vi "Display Float Values As Graph.vi"() -> ()   [LabVIEW 2014]
panel:
  out "Waveform Graph 2":dbl[](graph)
  out "Waveform Graph":dbl[](graph)
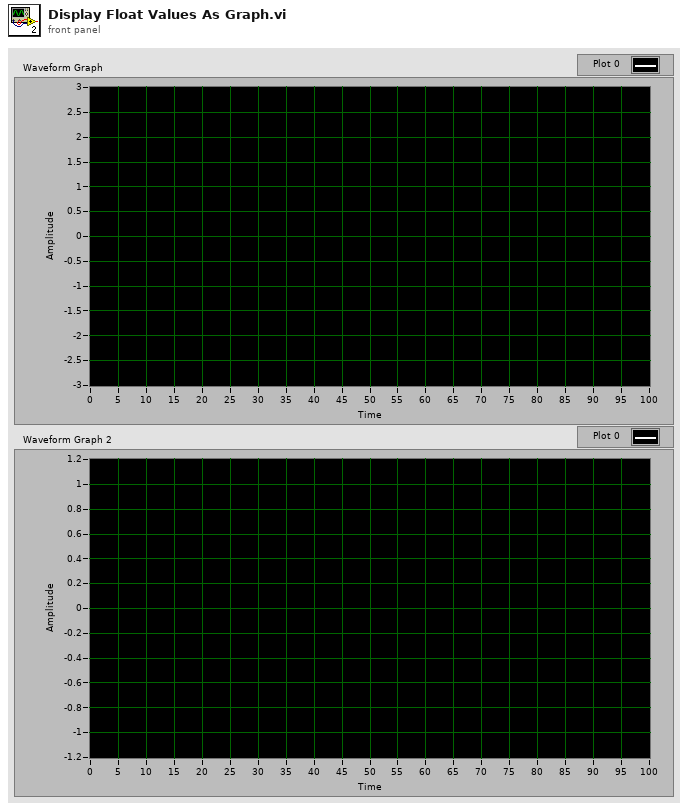
[diagram p1: front panel]
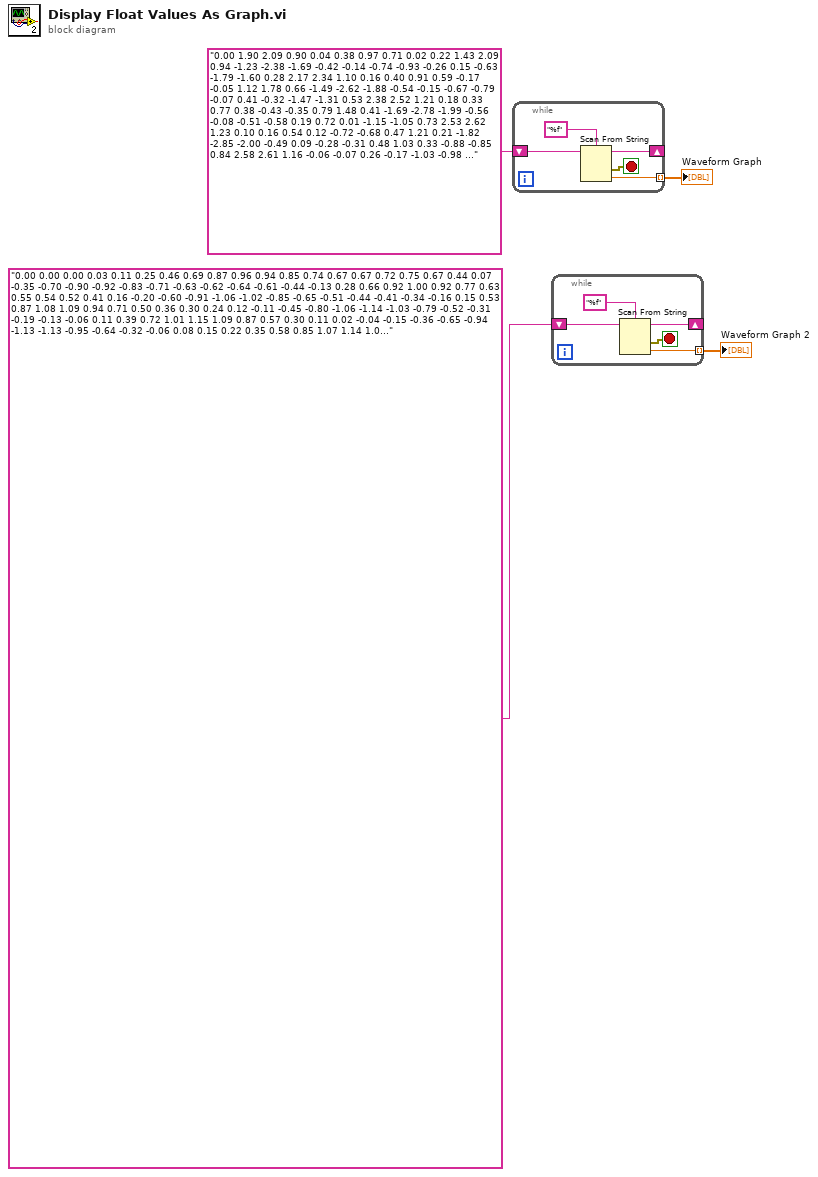
[diagram p0: block diagram]
diagram:
  n1 = while {
    shift-right: [w7] -> _
    shift-left: "0.00 1.90 2.09 0.90 0.04 0.38 0.97 0.71 0.02 0.22 1.43 2.09 0.94 -1.23 -2.38 -1.69 -0.42 -0.14 -0.74 -0.93 -0.26 0.15 -0.63 -1.79 -1.60 0.28 2.17 2.34 1.10 0.16 0.40 0.91 0.59 -0.17 -0.05 1.12 1.78 0.66 -1.49 -2.62 -1.88 -0.54 -0.15 -0.67 -0.79 -0.07 0.41 -0.32 -1.47 -1.31 0.53 2.38 2.52 1.21 0.18 0.33 0.77 0.38 -0.43 -0.35 0.79 1.48 0.41 -1.69 -2.78 -1.99 -0.56 -0.08 -0.51 -0.58 0.19 0.72 0.01 -1.15 -1.05 0.73 2.53 2.62 1.23 0.10 0.16 0.54 0.12 -0.72 -0.68 0.47 1.21 0.21 -1.82 -2.85 -2.00 -0.49 0.09 -0.28 -0.31 0.48 1.03 0.33 -0.88 -0.85 0.84 2.58 2.61 1.16 -0.06 -0.07 0.26 -0.17 -1.03 -0.98 0.19 1.01 0.10 -1.85 -2.83 -1.92 -0.33 0.32 0.01 -0.01 0.78 1.32 0.60 -0.67 -0.73 0.87 2.54 2.52 1.00 -0.29 -0.36 -0.04 -0.47 -1.31 -1.25 -0.02 0.88 0.07 -1.80 -2.72 -1.75 -0.10 0.61 0.32 0.29 1.06 1.57 0.81 -0.54 -0.70 0.80 2.41 2.34 0.77 -0.57 -0.68 -0.35 -0.75 -1.55 -1.44 -0.15 0.85 0.14 -1.65 -2.52 -1.52 0.18 0.92 0.63 0.57 1.29 1.75 0.93 -0.50 -0.77 0.64 2.19 2.09 0.49 -0.88 -0.99 -0.64 -0.97 -1.72 -1.55 -0.19 0.91 0.30 -1.42 -2.26 -1.24 0.47 1.23 0.92 0.80 1.44 1.84 0.96 -0.56 -0.93 0.41 1.91 1.80 0.20 -1.17 -1.27 -0.86 -1.12 -1.79 -1.56 -0.13 1.06 0.54 -1.12 -1.96 -0.95 0.76 1.50 1.14 0.95 1.51 1.84 0.89 -0.70 -1.16 0.11 1.60 1.50 -0.07 -1.43 -1.49 -1.01 -1.19 -1.78 -1.48 0.02 1.28 0.84 -0.80 -1.64 -0.67 1.00 1.70 1.29 1.01 1.48 1.75 0.73 -0.92 -1.45 -0.22 1.27 1.22 -0.31 -1.62 -1.63 -1.07 -1.15 -1.67 -1.31 0.24 1.56 1.16 -0.47 -1.35 -0.44 1.18 1.83 1.34 0.97 1.36 1.56 0.51 -1.19 -1.76 -0.55 0.97 0.99 -0.48 -1.73 -1.68 -1.03 -1.03 -1.47 -1.08 0.51 1.86 1.49 -0.16 -1.11 -0.28 1.28 1.87 1.30 0.84 1.16 1.31 0.24 -1.48 -2.07 -0.86 0.72 0.82 -0.56 -1.75 -1.63 -0.91 -0.82 -1.21 -0.80 0.80 2.16 1.79 0.10 -0.93 -0.19 1.28 1.80 1.17 0.64 0.89 1.02 -0.05 -1.77 -2.36 -1.11 0.54 0.74 -0.56 -1.67 -1.49 -0.70 -0.55 -0.91 -0.50 1.08 2.43 2.03 0.28 -0.84 -0.21 1.19 1.65 0.96 0.37 0.58 0.71 -0.34 -2.02 -2.58 -1.29 0.44 0.75 -0.45 -1.51 -1.27 -0.43 -0.24 -0.59 -0.21 1.32 2.64 2.19 0.37 -0.85 -0.32 1.01 1.43 0.70 0.06 0.26 0.42 -0.58 -2.22 -2.73 -1.38 0.45 0.85 -0.26 -1.27 -1.00 -0.13 0.08 -0.29 0.03 1.50 2.76 2.27 0.37 -0.95 -0.51 0.75 1.15 0.40 -0.25 -0.04 0.17 -0.76 -2.33 -2.79 -1.37 0.54 1.05 0.00 -0.97 -0.70 0.17 0.37 -0.04 0.22 1.60 2.80 2.25 0.28 -1.14 -0.77 0.45 0.84 0.10 -0.53 -0.29 -0.01 -0.85 -2.35 -2.75 -1.27 0.72 1.30 0.31 -0.66 -0.40 0.44 0.61 0.15 0.31 1.61 2.74 2.13 0.10 -1.39 -1.08 0.13 0.54 -0.17 -0.76 -0.47 -0.11 -0.86 -2.27 -2.61 -1.09 0.96 1.61 0.64 -0.35 -0.14 0.67 0.79 0.25 0.32 1.52 2.59 1.94 -0.14 -1.68 -1.41 -0.19 0.26 -0.38 -0.93 -0.56 -0.12 -0.76 -2.10 -2.40 -0.85 1.24 1.92 0.96 -0.07 0.08 0.82 0.87 0.25 0.22 1.35 2.36 1.69 -0.41 -1.98 -1.72 -0.47 0.05 -0.52 -1.00 -0.56 -0.03 -0.58 -1.86 -2.13 -0.57 1.53 2.22 1.24 0.15 0.21 0.87 0.86 0.16 0.04 1.09 2.07 1.40 -0.70 -2.27 -2.00 -0.69 -0.09 -0.57 -0.97 -0.47 0.15 -0.33 -1.56 -1.84 -0.29 1.81 2.48 1.45 0.29 0.26 0.84 0.76 -0.02 -0.21 0.79 1.76 1.11 -0.96 -2.51 -2.20 -0.83 -0.13 -0.52 -0.86 -0.29 0.39 -0.03 -1.24 -1.53 -0.03 2.03 2.68 1.59 0.33 0.20 0.71 0.57 -0.26 -0.50 0.46 1.45 0.85 -1.17 -2.69 -2.33 -0.88 -0.08 -0.39 -0.66 -0.04 0.68 0.30 -0.92 -1.26 0.19 2.19 2.78 1.63 0.28 0.06 0.50 0.32 -0.55 -0.82 0.14 1.16 0.63 -1.32 -2.77 -2.36 -0.83 0.07 -0.17 -0.39 0.24 0.99 0.62 -0.63 -1.04 0.32 2.26 2.80 1.58 0.14 -0.16 0.23 0.02 -0.85 -1.13 -0.15 0.94 0.49 -1.37 -2.77 -2.29 -0.69 0.28 0.11 -0.09 0.54 1.29 0.90 -0.40 -0.89 0.37 2.23 2.71 1.43 -0.07 -0.44 -0.08 -0.28 -1.14 -1.40 -0.38 0.78 0.44 -1.33 -2.66 -2.14 -0.47 0.56 0.42 0.22 0.83 1.55 1.12 -0.24 -0.84 0.33 2.11 2.54 1.22 -0.34 -0.75 -0.40 -0.57 -1.38 -1.60 -0.53 0.72 0.49 -1.20 -2.48 -1.91 -0.21 0.86 0.74 0.51 1.07 1.74 1.26 -0.18 -0.88 0.19 1.91 2.30 0.95 -0.64 -1.06 -0.69 -0.81 -1.56 -1.73 -0.58 0.76 0.63 -0.98 -2.22 -1.64 0.08 1.17 1.03 0.75 1.24 1.85 1.30 -0.21 -1.01 -0.03 1.63 2.02 0.66 -0.93 -1.35 -0.93 -0.98 -1.66 -1.76 -0.54 0.89 0.84 -0.70 -1.92 -1.35 0.37 1.44 1.27 0.92 1.33 1.86 1.25 -0.34 -1.22 -0.32 1.32 1.71 0.38 -1.20 -1.58 -1.10 -1.06 -1.66 -1.69 -0.42 1.09 1.12 -0.38 -1.60 -1.06 0.62 1.66 1.44 1.00 1.32 1.78 1.11 -0.54 -1.49 -0.64 0.99 1.42 0.13 -1.40 -1.73 -1.18 -1.05 -1.57 -1.54 -0.21 1.35 1.44 -0.04 -1.29 -0.81 0.81 1.80 1.51 0.99 1.22 1.61 0.90 -0.80 -1.80 -0.97 0.68 1.16 -0.05 -1.53 -1.80 -1.17 -0.95 -1.38 -1.31 0.05 1.65 1.76 0.28 -1.03 -0.63 0.92 1.85 1.49 0.88 1.03 1.37 0.63 -1.08 -2.11 -1.29 0.41 0.97 -0.16 -1.56 -1.77 -1.06 -0.76 -1.13 -1.03 0.34 1.94 2.06 0.55 -0.83 -0.52 0.94 1.81 1.38 0.70 0.78 1.08 0.34 -1.37 -2.39 -1.55 0.20 0.87 -0.17 -1.50 -1.65 -0.87 -0.50 -0.83 -0.73 0.62 2.21 2.31 0.75 -0.72 -0.51 0.87 1.67 1.19 0.44 0.48 0.77 0.05 -1.63 -2.63 -1.74 0.08 0.85 -0.09 -1.35 -1.44 -0.62 -0.20 -0.52 -0.43 0.88 2.43 2.49 0.86 -0.70 -0.60 0.70 1.46 0.93 0.15 0.16 0.46 -0.21 -1.84 -2.78 -1.85 0.06 0.93 0.09 -1.12 -1.18 -0.33 0.11 -0.21 -0.17 1.07 2.57 2.58 0.89 -0.77 -0.77 0.46 1.18 0.64 -0.16 -0.15 0.20 -0.41 -1.96 -2.85 -1.86 0.13 1.10 0.33 -0.83 -0.88 -0.03 0.41 0.06 0.03 1.19 2.62 2.58 0.81 -0.93 -1.02 0.16 0.87 0.34 -0.45 -0.41 -0.01 -0.52 -2.00 -2.83 -1.78 0.29 1.34 0.64 -0.51 -0.58 0.25 0.66 0.26 0.15 1.22 2.58 2.48 0.65 -1.16 -1.31 -0.16 0.56 0.06 -0.69 -0.61 -0.13 -0.55 -1.94 -2.71 -1.61 0.51 1.63 0.96 -0.19 -0.30 0.49 0.85 0.38 0.18 1.15 2.44 2.29 0.43 -1.44 -1.63 -0.48 0.28 -0.17 -0.87 -0.72 -0.16 -0.48 -1.79 -2.51 -1.38 0.79 1.94 1.28 0.10 -0.07 0.65 0.95 0.41 0.11 1.00 2.22 2.04 0.16 -1.74 -1.95 -0.78 0.04 -0.33 -0.96 -0.74 -0.09 -0.32 -1.56 -2.24 -1.10 1.07 2.24 1.57 0.34 0.09 0.73 0.96 0.34 -0.05 0.76 1.94 1.76 -0.13 -2.03 -2.23 -1.02 -0.12 -0.40 -0.95 -0.66 0.06 -0.09 -1.27 -1.94 -0.81 1.35 2.50 1.81 0.50 0.15 0.71 0.87 0.18 -0.28 0.47 1.62 1.46 -0.40 -2.28 -2.45 -1.18 -0.18 -0.37 -0.85 -0.50 0.29 0.20 -0.94 -1.63 -0.54 1.58 2.71 1.96 0.57 0.13 0.60 0.70 -0.05 -0.56 0.14 1.30 1.18 -0.62 -2.46 -2.59 -1.24 -0.16 -0.25 -0.66 -0.27 0.57 0.52 -0.62 -1.34 -0.32 1.75 2.83 2.02 0.54 0.01 0.40 0.46 -0.32 -0.87 -0.18 1.01 0.95 -0.78 -2.56 -2.63 -1.22 -0.04 -0.05 -0.41 0.02 0.87 0.84 -0.32 -1.10 -0.16 1.83 2.85 1.98 0.42 -0.20 0.14 0.17 -0.63 -1.18 -0.48 0.76 0.79 -0.86 -2.57 -2.58 -1.10 0.16 0.22 -0.11 0.32 1.17 1.13 -0.07 -0.93 -0.09 1.83 2.79 1.86 0.23 -0.46 -0.16 -0.14 -0.92 -1.46 -0.72 0.58 0.71 -0.84 -2.48 -2.44 -0.90 0.42 0.52 0.20 0.61 1.44 1.36 0.11 -0.85 -0.11 1.72 2.63 1.66 -0.03 -0.77 -0.48 -0.44 -1.17 -1.67 -0.89 0.50 0.73 -0.72 -2.30 -2.23 -0.65 0.72 0.84 0.50 0.86 1.64 1.51 0.19 -0.86 -0.22 1.53 2.39 1.40 -0.32 -1.08 -0.78 -0.69 -1.37 -1.81 -0.96 0.51 0.84 -0.52 -2.05 -1.96 -0.36 1.02 1.14 0.76 1.05 1.76 1.57 0.18 -0.97" -> [w9]
    tunnel: [w5] -> w3 mode=indexing
    stop <- w6 stop-if-true
    n2 = Scan From String(format string="%f", input string=w9) -> (remaining string=w7:string, error out=w6:errorcluster, output 1=w5:dbl)  [unwired: 3 in, 1 out]
  }
  "Waveform Graph" <- w3
  n3 = while {
    shift-right: [w12] -> _
    shift-left: "0.00 0.00 0.00 0.03 0.11 0.25 0.46 0.69 0.87 0.96 0.94 0.85 0.74 0.67 0.67 0.72 0.75 0.67 0.44 0.07 -0.35 -0.70 -0.90 -0.92 -0.83 -0.71 -0.63 -0.62 -0.64 -0.61 -0.44 -0.13 0.28 0.66 0.92 1.00 0.92 0.77 0.63 0.55 0.54 0.52 0.41 0.16 -0.20 -0.60 -0.91 -1.06 -1.02 -0.85 -0.65 -0.51 -0.44 -0.41 -0.34 -0.16 0.15 0.53 0.87 1.08 1.09 0.94 0.71 0.50 0.36 0.30 0.24 0.12 -0.11 -0.45 -0.80 -1.06 -1.14 -1.03 -0.79 -0.52 -0.31 -0.19 -0.13 -0.06 0.11 0.39 0.72 1.01 1.15 1.09 0.87 0.57 0.30 0.11 0.02 -0.04 -0.15 -0.36 -0.65 -0.94 -1.13 -1.13 -0.95 -0.64 -0.32 -0.06 0.08 0.15 0.22 0.35 0.58 0.85 1.07 1.14 1.01 0.72 0.36 0.05 -0.16 -0.26 -0.31 -0.38 -0.54 -0.77 -0.99 -1.11 -1.04 -0.79 -0.43 -0.06 0.22 0.37 0.42 0.45 0.53 0.70 0.90 1.04 1.04 0.85 0.50 0.11 -0.23 -0.45 -0.53 -0.54 -0.56 -0.65 -0.81 -0.96 -1.00 -0.87 -0.57 -0.17 0.22 0.50 0.63 0.64 0.62 0.64 0.73 0.86 0.93 0.86 0.62 0.24 -0.17 -0.51 -0.70 -0.75 -0.71 -0.66 -0.68 -0.76 -0.84 -0.82 -0.64 -0.31 0.11 0.49 0.75 0.85 0.81 0.72 0.66 0.68 0.73 0.75 0.63 0.36 -0.04 -0.45 -0.76 -0.92 -0.91 -0.80 -0.68 -0.62 -0.63 -0.65 -0.58 -0.38 -0.03 0.38 0.74 0.96 1.00 0.89 0.73 0.60 0.54 0.54 0.50 0.36 0.08 -0.31 -0.69 -0.96 -1.06 -0.99 -0.80 -0.61 -0.48 -0.43 -0.40 -0.31 -0.09 0.24 0.62 0.94 1.10 1.07 0.89 0.65 0.45 0.34 0.29 0.23 0.08 -0.19 -0.54 -0.88 -1.10 -1.13 -0.98 -0.72 -0.46 -0.27 -0.18 -0.12 -0.03 0.17 0.47 0.81 1.06 1.15 1.05 0.80 0.50 0.24 0.08 0.01 -0.06 -0.19 -0.42 -0.72 -1.00 -1.14 -1.10 -0.88 -0.56 -0.24 -0.01 0.10 0.16 0.24 0.40 0.65 0.92 1.10 1.12 0.95 0.64 0.28 -0.02 -0.20 -0.28 -0.32 -0.41 -0.59 -0.83 -1.03 -1.11 -0.99 -0.71 -0.34 0.02 0.27 0.39 0.42 0.46 0.57 0.75 0.95 1.06 1.01 0.77 0.41 0.01 -0.30 -0.48 -0.53 -0.54 -0.58 -0.69 -0.85 -0.98 -0.98 -0.81 -0.48 -0.07 0.30 0.54 0.64 0.64 0.62 0.66 0.77 0.89 0.93 0.82 0.54 0.14 -0.27 -0.58 -0.73 -0.74 -0.69 -0.66 -0.70 -0.79 -0.85 -0.79 -0.57 -0.21 0.21 0.57 0.79 0.85 0.78 0.70 0.66 0.69 0.74 0.73 0.58 0.27 -0.14 -0.54 -0.82 -0.93 -0.89 -0.76 -0.66 -0.62 -0.64 -0.64 -0.54 -0.30 0.07 0.48 0.81 0.99 0.98 0.85 0.69 0.58 0.54 0.53 0.48 0.30 -0.01 -0.40 -0.77 -1.01 -1.06 -0.95 -0.75 -0.57 -0.46 -0.42 -0.39 -0.27 -0.02 0.33 0.71 0.99 1.11 1.03 0.83 0.59 0.42 0.32 0.28 0.20 0.02 -0.27 -0.63 -0.95 -1.12 -1.11 -0.92 -0.65 -0.40 -0.24 -0.16 -0.10 0.02 0.24 0.56 0.88 1.10 1.15 1.00 0.72 0.42 0.19 0.06 -0.01 -0.08 -0.24 -0.49 -0.80 -1.05 -1.15 -1.06 -0.81 -0.47 -0.17 0.02 0.12 0.18 0.27 0.46 0.72 0.97 1.13 1.10 0.88 0.54 0.19 -0.08 -0.22 -0.29 -0.34 -0.45 -0.65 -0.89 -1.07 -1.10 -0.94 -0.62 -0.24 0.09 0.31 0.40 0.43 0.48 0.61 0.80 0.98 1.06 0.97 0.69 0.31 -0.08 -0.36 -0.50 -0.54 -0.54 -0.60 -0.73 -0.89 -1.00 -0.96 -0.74 -0.38 0.03 0.37 0.58 0.64 0.63 0.62 0.68 0.80 0.90 0.92 0.77 0.45 0.04 -0.36 -0.63 -0.74 -0.73 -0.68 -0.66 -0.72 -0.80 -0.84 -0.75 -0.50 -0.11 0.31 0.64 0.82 0.84 0.76 0.68 0.66 0.71 0.75 0.71 0.51 0.17 -0.24 -0.62 -0.86 -0.93 -0.86 -0.73 -0.64 -0.62 -0.64 -0.63 -0.50 -0.22 0.17 0.57 0.87 1.00 0.96 0.81 0.66 0.56 0.54 0.53 0.45 0.24 -0.10 -0.50 -0.85 -1.04 -1.04 -0.90 -0.70 -0.54 -0.45 -0.42 -0.36 -0.22 0.06 0.43 0.79 1.04 1.11 0.99 0.77 0.54 0.39 0.31 0.26 0.17 -0.04 -0.36 -0.72 -1.01 -1.14 -1.07 -0.85 -0.58 -0.36 -0.22 -0.15 -0.08 0.06 0.31 0.64 0.95 1.13 1.13 0.94 0.65 0.36 0.15 0.04 -0.02 -0.11 -0.29 -0.57 -0.87 -1.09 -1.15 -1.01 -0.72 -0.39 -0.12 0.06 0.14 0.19 0.31 0.52 0.78 1.03 1.14 1.06 0.80 0.45 0.12 -0.12 -0.25 -0.30 -0.36 -0.49 -0.71 -0.94 -1.09 -1.08 -0.87 -0.53 -0.15 0.16 0.34 0.41 0.44 0.50 0.65 0.85 1.02 1.06 0.91 0.60 0.21 -0.16 -0.40 -0.52 -0.54 -0.55 -0.62 -0.77 -0.93 -1.00 -0.92 -0.66 -0.28 0.12 0.44 0.61 0.65 0.63 0.63 0.70 0.83 0.92 0.90 0.70 0.35 -0.07 -0.44 -0.67 -0.75 -0.72 -0.67 -0.67 -0.74 -0.82 -0.84 -0.70 -0.41 -0.00 0.40 0.70 0.84 0.83 0.74 0.67 0.67 0.72 0.75 0.67 0.44 0.07 -0.35 -0.70 -0.89 -0.92 -0.83 -0.71 -0.63 -0.62 -0.65 -0.61 -0.44 -0.13 0.28 0.66 0.92 1.00 0.93 0.77 0.62 0.55 0.54 0.52 0.41 0.16 -0.21 -0.60 -0.91 -1.05 -1.02 -0.85 -0.65 -0.50 -0.44 -0.41 -0.34 -0.16 0.15 0.53 0.87 1.07 1.09 0.94 0.71 0.50 0.36 0.30 0.25 0.13 -0.11 -0.45 -0.80 -1.06 -1.14 -1.03 -0.79 -0.52 -0.31 -0.19 -0.14 -0.06 0.11 0.39 0.72 1.01 1.15 1.09 0.87 0.57 0.30 0.11 0.02 -0.04 -0.15 -0.36 -0.65 -0.94 -1.12 -1.13 -0.95 -0.64 -0.32 -0.06 0.08 0.15 0.21 0.35 0.58 0.85 1.07 1.14 1.01 0.72 0.37 0.05 -0.17 -0.26 -0.31 -0.38 -0.54 -0.77 -0.99 -1.10 -1.04 -0.80 -0.43 -0.06 0.22 0.37 0.42 0.45 0.53 0.70 0.90 1.04 1.04 0.85 0.51 0.11 -0.23 -0.45 -0.53 -0.54 -0.56 -0.65 -0.81 -0.96 -1.00 -0.87 -0.58 -0.18 0.21 0.50 0.63 0.64 0.62 0.64 0.73 0.86 0.93 0.86 0.62 0.25 -0.17 -0.51 -0.71 -0.75 -0.71 -0.66 -0.68 -0.76 -0.84 -0.82 -0.64 -0.31 0.10 0.49 0.75 0.85 0.81 0.72 0.66 0.68 0.73 0.74 0.63 0.36 -0.03 -0.44 -0.76 -0.92 -0.91 -0.80 -0.68 -0.62 -0.63 -0.65 -0.58 -0.38 -0.03 0.37 0.74 0.96 1.00 0.89 0.73 0.60 0.54 0.54 0.50 0.36 0.08 -0.30 -0.69 -0.96 -1.06 -0.99 -0.80 -0.61 -0.48 -0.43 -0.40 -0.31 -0.09 0.24 0.62 0.93 1.10 1.07 0.89 0.65 0.45 0.34 0.29 0.23 0.08 -0.19 -0.54 -0.88 -1.10 -1.13 -0.98 -0.72 -0.46 -0.27 -0.18 -0.12 -0.02 0.17 0.47 0.80 1.06 1.16 1.05 0.80 0.50 0.24 0.08 0.01 -0.06 -0.19 -0.42 -0.72 -1.00 -1.15 -1.11 -0.88 -0.56 -0.24 -0.02 0.10 0.16 0.24 0.40 0.65 0.91 1.10 1.12 0.95 0.64 0.28 -0.02 -0.20 -0.27 -0.32 -0.42 -0.59 -0.83 -1.03 -1.11 -1.00 -0.71 -0.34 0.02 0.26 0.38 0.42 0.46 0.57 0.75 0.94 1.06 1.01 0.78 0.41 0.01 -0.30 -0.48 -0.53 -0.54 -0.58 -0.69 -0.85 -0.98 -0.99 -0.82 -0.48 -0.07 0.30 0.54 0.64 0.64 0.62 0.66 0.76 0.88 0.93 0.82 0.54 0.14 -0.27 -0.58 -0.73 -0.74 -0.69 -0.66 -0.70 -0.78 -0.84 -0.79 -0.58 -0.21 0.21 0.57 0.79 0.84 0.78 0.70 0.66 0.69 0.74 0.73 0.58 0.27 -0.14 -0.54 -0.82 -0.93 -0.88 -0.76 -0.66 -0.62 -0.64 -0.64 -0.54 -0.30 0.07 0.48 0.81 0.98 0.98 0.85 0.69 0.58 0.54 0.53 0.48 0.30 -0.01 -0.40 -0.77 -1.01 -1.06 -0.94 -0.75 -0.57 -0.46 -0.42 -0.38 -0.27 -0.02 0.33 0.71 0.99 1.11 1.03 0.83 0.60 0.42 0.32 0.27 0.20 0.02 -0.27 -0.63 -0.95 -1.12 -1.10 -0.92 -0.65 -0.41 -0.24 -0.16 -0.10 0.01 0.24 0.55 0.88 1.10 1.15 1.00 0.72 0.43 0.19 0.06 -0.01 -0.08 -0.24 -0.49 -0.80 -1.05 -1.15 -1.06 -0.81 -0.48 -0.18 0.02 0.12 0.18 0.27 0.45 0.71 0.97 1.13 1.10 0.88 0.55 0.20 -0.07 -0.22 -0.29 -0.34 -0.45 -0.65 -0.89 -1.07 -1.10 -0.94 -0.62 -0.24 0.09 0.30 0.40 0.43 0.48 0.61 0.80 0.98 1.06 0.97 0.69 0.31 -0.07 -0.36 -0.50 -0.54 -0.54 -0.60 -0.72 -0.89 -1.00 -0.96 -0.74 -0.38 0.03 0.37 0.58 0.65 0.63 0.62 0.68 0.79 0.91 0.92 0.77 0.45 0.04 -0.35 -0.63 -0.74 -0.73 -0.68 -0.66 -0.71 -0.80 -0.85 -0.76 -0.50 -0.11 0.31 0.64 0.82 0.84 0.76 0.68 0.66 0.70 0.75 0.71 0.51 0.17 -0.24 -0.62 -0.86 -0.93 -0.86 -0.74 -0.64 -0.62 -0.64 -0.63 -0.50 -0.22 0.17" -> [w14]
    tunnel: [w10] -> w2 mode=indexing
    stop <- w11 stop-if-true
    n4 = Scan From String(format string="%f", input string=w14) -> (remaining string=w12:string, error out=w11:errorcluster, output 1=w10:dbl)  [unwired: 3 in, 1 out]
  }
  "Waveform Graph 2" <- w2
